vi "AskToMotor.vi"(8 "error in (no error)":errorcluster, 9 "Período":sgl, 10 "MG17Piezo":refnum<k7>, 11 "amplitude":sgl) -> (0 "error out":errorcluster)   [LabVIEW 2014]
panel:
  out "abs(x)":sgl
  in  "pfVoltage":sgl
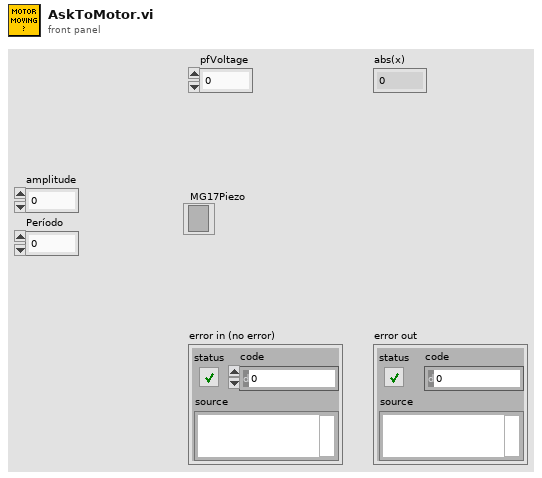
[diagram p1: front panel]
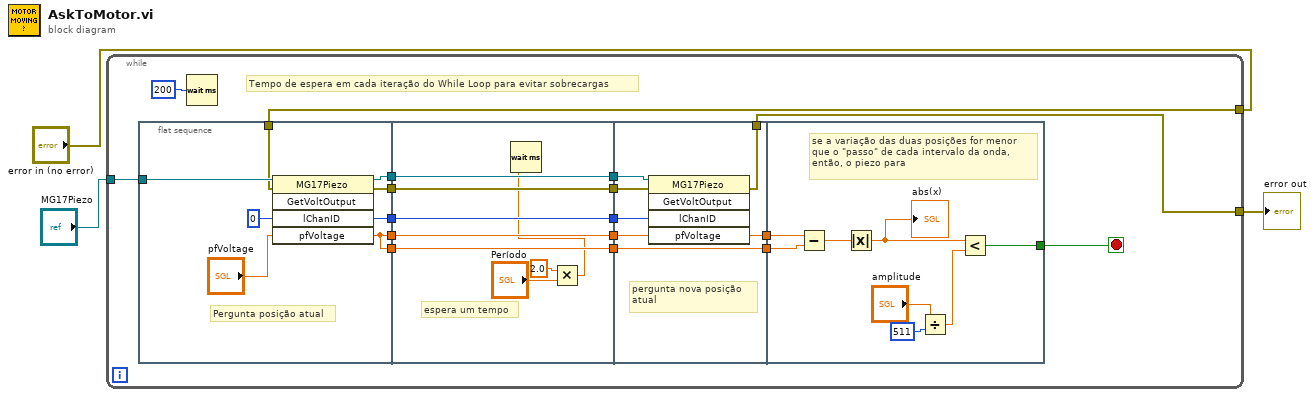
[diagram p0: block diagram]
diagram:
  n1 = while {
    tunnel: "MG17Piezo" -> [w11]
    tunnel: [w5] -> w2
    tunnel: "error in (no error)" -> [w4]
    stop <- w12 stop-if-true
    # "Tempo de espera em cada iteração do While Loop para evitar sobrecargas"
    n2 = flat-sequence {
      tunnel: [w28] -> w19
      tunnel: [w27] -> w17
      tunnel: [w23] -> w13
      tunnel: w11 -> [w26]
      tunnel: [w23] -> w8
      tunnel: [w22] -> w6
      tunnel: w4 -> [w21]
      tunnel: [w36] -> w20
      tunnel: w19 -> [w36]
      tunnel: [w35] -> w18
      tunnel: w17 -> [w35]
      tunnel: [w34] -> w14
      tunnel: w13 -> [w34]
      tunnel: [w33] -> w9
      tunnel: w8 -> [w33]
      tunnel: [w32] -> w7
      tunnel: w6 -> [w32]
      tunnel: w20 -> [w43]
      tunnel: w18 -> [w42]
      tunnel: [w41] -> w16
      tunnel: [w40] -> w15
      tunnel: w14 -> [w40]
      tunnel: w9 -> [w39]
      tunnel: w7 -> [w38]
      tunnel: [w37] -> w5
      tunnel: w16 -> [w51]
      tunnel: w15 -> [w50]
      tunnel: [w49] -> w12
      frame #0 {
        # "Pergunta posição atual"
        n3 = invoke class="MG17Piezo" method="GetVoltOutput"(reference=w26, error in=w21, "lChanID"=0, "pfVoltage"="pfVoltage") -> (reference out=w28:refnum<k7>, error out=w22:errorcluster, "lChanID"=w27:i32, "pfVoltage"=w23:sgl)  [unwired: 1 in, 1 out]
      }
      frame #1 {
        # "espera um tempo"
        n4 = Multiply(x=sgl 2.0, y="Período") -> (x*y=w30:sgl)
        n5 = Wait (ms)(milliseconds to wait=w30) -> ()  [unwired: 1 out]
      }
      frame #2 {
        # "pergunta nova posição \natual"
        n6 = invoke class="MG17Piezo" method="GetVoltOutput"(reference=w43, error in=w38, "lChanID"=w42, "pfVoltage"=w39) -> (error out=w37:errorcluster, "pfVoltage"=w41:sgl)  [unwired: 1 in, 3 out]
      }
      frame #3 {
        # "se a variação das duas posições for menor \nque o \"passo\" de cada intervalo da onda,\nentão, o piezo para"
        n7 = Subtract(x=w51, y=w50) -> (x-y=w48:sgl)
        n8 = Absolute Value(x=w48) -> (abs(x)=w47:sgl)
        "abs(x)" <- w47
        n9 = Divide(x="amplitude", y=511) -> (x/y=w45:sgl)
        n10 = Less?(x=w47, y=w45) -> (x < y?=w49:bool)
      }
    }
    n11 = Wait (ms)(milliseconds to wait=u32 200) -> ()  [unwired: 1 out]
  }
  "error out" <- w2
